vi "Update from Module Class.vi"(8 "error in":errorcluster, 9 "module in":refnum<class "Module.lvclass">, 10 "slot ref in":T1=18446744073709551615 format="%.0x", 11 "RSI Module in":refnum<class "RSI Module.lvclass">) -> (0 "error out":errorcluster, 1 "module out":refnum<class "Module.lvclass">, 2 "slot ref out":T1=18446744073709551615 format="%.0x", 3 "RSI Module out":refnum<class "RSI Module.lvclass">)   [LabVIEW 2017, in "Modules.lvlib" / "RSI Module.lvclass"]
uses:
  RSI Module.lvclass
  niveristand-scan-engine-ethercat-custom-device/Custom Device Source/Scripting/Modules/Module/Module.lvclass
  <vilib>/NI Veristand/Custom Device API/Custom Device Item Ref.ctl
  <vilib>/NI Veristand/Custom Device API/Custom Device API.lvlib
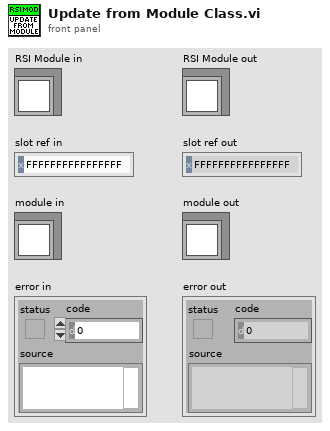
[diagram p1: front panel]
types:
  T1 = typedef "Custom Device API.lvlib/Custom Device Item Ref.ctl" = u64
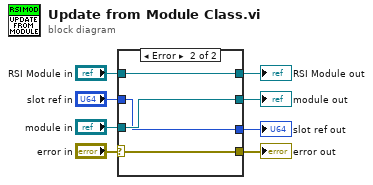
[diagram p0: block diagram]
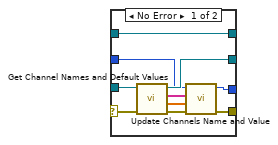
[diagram p2: hidden frame]
diagram:
  n1 = case shown="Error" "error in" {
    selector: "error in" -> [w13 w22]
    tunnel: [w17 w22] -> w7
    tunnel: [w18 w21] -> w5
    tunnel: "RSI Module in" -> [w18 w21]
    tunnel: "module in" -> [w16 w20]
    tunnel: [w12 w20] -> w3
    tunnel: [w10 w19] -> w2
    tunnel: "slot ref in" -> [w9 w19]
    frame No Error {
      n2 = call-dynamic "Get Channel Names and Default Values.vi"("error in"=w13, "module in"=w16) -> ("error out"=w11:errorcluster, "default values"=w14:dbl[], "names"=w15:string[], "module out"=w12:refnum<class "Module.lvclass">)  [unwired: 6 in]
      n3 = call "Update Channels Name and Value.vi"("error in"=w11, "default values"=w14, "channel names"=w15, "slot ref in"=w9) -> ("error out"=w17:errorcluster, "slot ref out"=w10:T1)  [unwired: 6 in]
    }
    frame Error {
    }
  }
  "error out" <- w7
  "RSI Module out" <- w5
  "module out" <- w3
  "slot ref out" <- w2
